vi "EvaluatePoint.vi"(8 "error in (no error)":errorcluster, 9 "GameRef":refnum<data-value>, 10 "Point":dbl[](array[numeric]), 11 "SupportAttackerPosition in":refnum<class "SupportAttackerPosition.lvclass">) -> (0 "error out":errorcluster, 2 "Evaluation":dbl, 3 "SupportAttackerPosition out":refnum<class "SupportAttackerPosition.lvclass">)   [LabVIEW 2023, in "SupportAttackerPosition.lvclass"]
uses:
  SupportAttackerPosition.lvclass
  Game_class/Game.lvclass
  Evaluator_class/Evaluator.lvclass
  SupportAttackerPosition.lvclass/SupportAttackerPosition.ctl
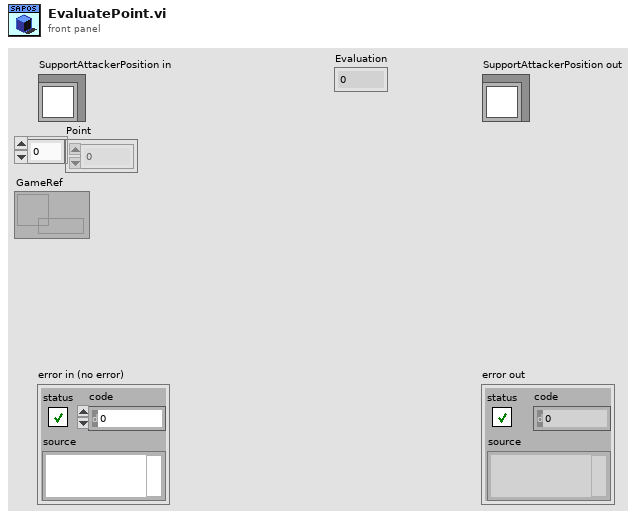
[diagram p1: front panel]
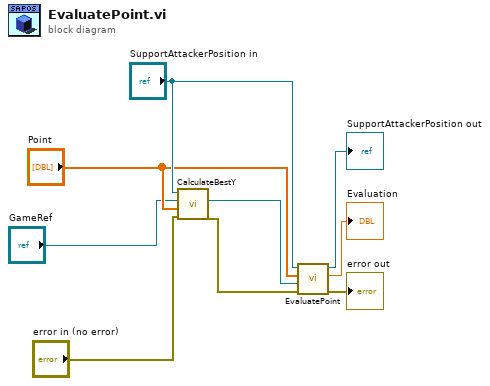
[diagram p0: block diagram]
diagram:
  n1 = call-dynamic "CalculateBestY.vi"("error in (no error)"="error in (no error)", "Point"="Point", "GameRef in"="GameRef", "SupportAttackerPosition in"="SupportAttackerPosition in") -> ("error out"=w3:errorcluster, "GameRef out"=w2:refnum<data-value>)  [unwired: 5 in, 1 out]
  n2 = call-parent "EvaluatePoint.vi"("error in (no error)"=w3, "GameRef"=w2, "Point"="Point", "Evaluator in"="SupportAttackerPosition in") -> ("error out"=→"error out":errorcluster, "Evaluation"=→"Evaluation":dbl, "Evaluator out"=→"SupportAttackerPosition out":refnum<class "SupportAttackerPosition.lvclass">)  [unwired: 5 in]
